vi "Set Token.vi"(4 "Sync Token Refnum":T1) -> ()   [LabVIEW 2019, in "Sync Token.lvlib"]
doc: "Signals a <b>Sync Token</b>, releasing any code that is currently waiting on it via <b>Wait on Token.vi</b>. This VI completes the synchronisation by sending a notification through the token's underlying Notifier, effectively \"setting\" the token."
uses:
  Controls/Public/Sync Token Refnum.ctl
  Sync Token.lvlib
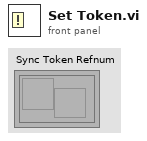
[diagram p1: front panel]
types:
  T1 = typedef "Sync Token.lvlib/Sync Token Refnum.ctl" = refnum<k1>
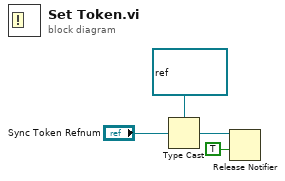
[diagram p0: block diagram]
diagram:
  n1 = Type Cast(type=refnum<notifier> refnum ("notifier out"), x="Sync Token Refnum") -> (*(type *) &x=w2:refnum<notifier>)
  n2 = Release Notifier(notifier=w2, force destroy? (F)=TRUE) -> ()  [unwired: 1 in, 3 out]
